vi "updateM300NTCENTwithPeeling.vi"() -> ()   [LabVIEW 2012]
uses:
  <vilib>/addons/database/Connection.llb/DB Tools Open Connec (Path).vi
  <vilib>/addons/database/Connection.llb/Conn Execute.vi
  <vilib>/addons/database/Recordset.llb/Rec Destroy - Connection.vi
  <vilib>/addons/database/Recordset.llb/Rec Fetch Recordset Data (R).vi
  <vilib>/addons/database/_DB Variant To Data/Database Variant To Data.xnode
  <vilib>/addons/database/NI_Database_API.lvlib
panel:
  out "concatenated string":string
  out "error out":errorcluster
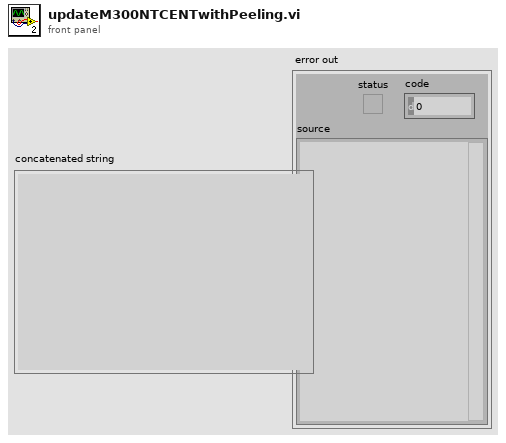
[diagram p1: front panel]
types:
  T1 = typedef "NI_Database_API.lvlib/Conn ObjectReference.ctl" = refnum<k1>
  T2 = typedef "NI_Database_API.lvlib/Rec ObjectReference.ctl" = refnum<k1>
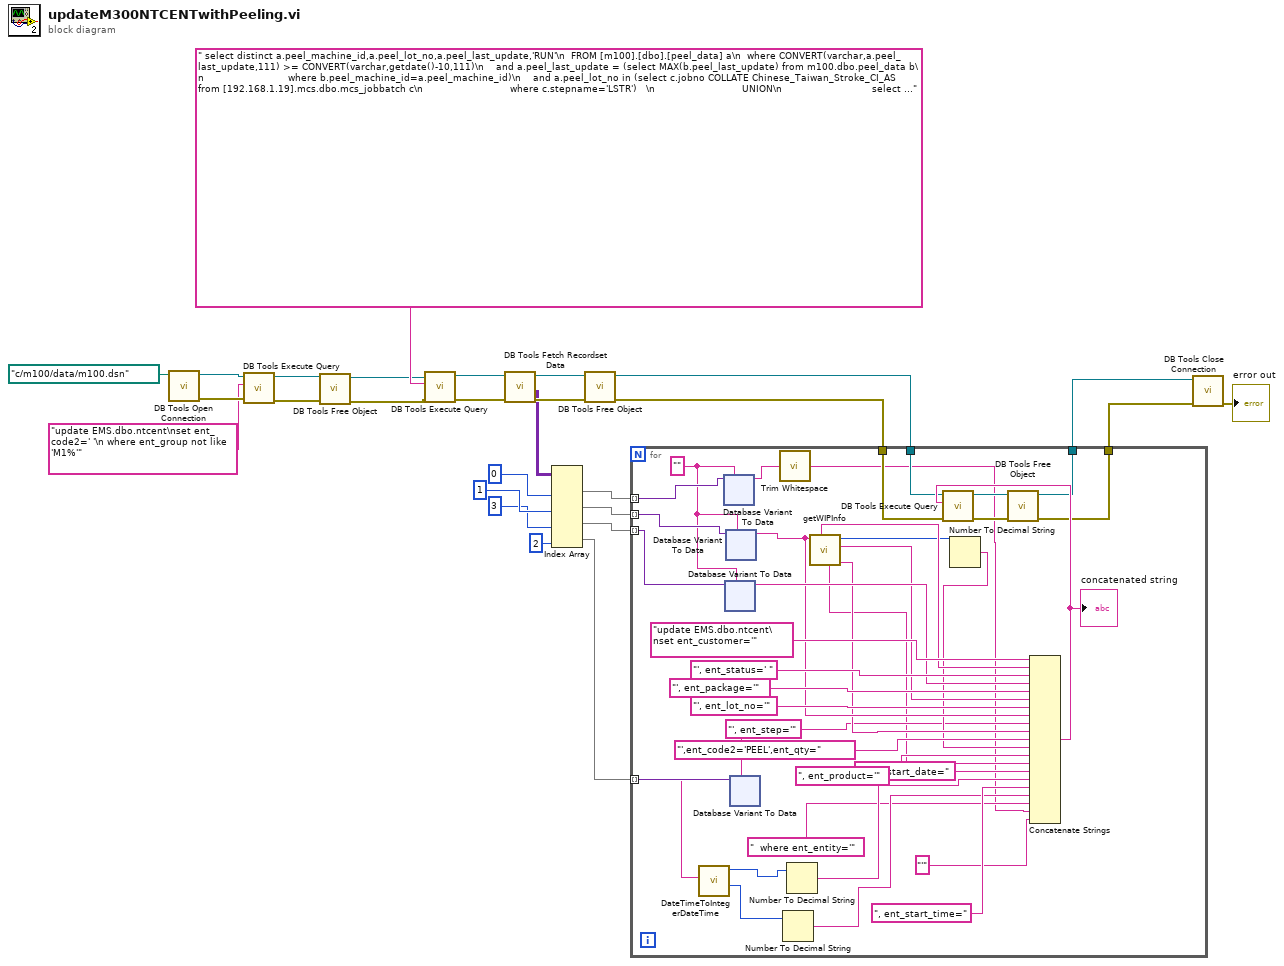
[diagram p0: block diagram]
diagram:
  n1 = call-poly <vilib>:"DB Tools Open Connection.vi"("connection information"=path "c:/m100/data/m100.dsn") -> ("error out"=w4:errorcluster, "connection reference"=w7:T1)  [unwired: 7 in]
  n2 = call-poly <vilib>:"DB Tools Execute Query.vi"("error in (no error)"=w4, "SQL query"="update EMS.dbo.ntcent\nset ent_code2=' '\n where ent_group not like 'M1%'", "connection reference"=w7) -> ("error out"=w3:errorcluster, "recordset reference"=w6:T2)  [unwired: 5 in]
  n3 = call-poly <vilib>:"DB Tools Free Object.vi"("error in (no error)"=w3, "recordset reference"=w6) -> ("error out"=w2:errorcluster, "connection reference"=w5:T1)  [unwired: 8 in]
  n4 = call-poly <vilib>:"DB Tools Execute Query.vi"("error in (no error)"=w2, "SQL query"=" select distinct a.peel_machine_id,a.peel_lot_no,a.peel_last_update,'RUN'\n  FROM [m100].[dbo].[peel_data] a\n  where CONVERT(varchar,a.peel_last_update,111) >= CONVERT(varchar,getdate()-10,111)\n    and a.peel_last_update = (select MAX(b.peel_last_update) from m100.dbo.peel_data b\n                            where b.peel_machine_id=a.peel_machine_id)\n    and a.peel_lot_no in (select c.jobno COLLATE Chinese_Taiwan_Stroke_CI_AS from [192.168.1.19].mcs.dbo.mcs_jobbatch c\n                             where c.stepname='LSTR')   \n                             UNION\n                              select distinct a.peel_machine_id,a.peel_lot_no,a.peel_last_update,'IDLE'\n  FROM [m100].[dbo].[peel_data] a\n  where CONVERT(varchar,a.peel_last_update,111) >= CONVERT(varchar,getdate()-10,111)\n    and a.peel_last_update = (select MAX(b.peel_last_update) from m100.dbo.peel_data b\n                            where b.peel_machine_id=a.peel_machine_id)\n    and a.peel_lot_no NOT in (select c.jobno COLLATE Chinese_Taiwan_Stroke_CI_AS from [192.168.1.19].mcs.dbo.mcs_jobbatch c\n                             where c.stepname='LSTR')  \n  order by a.peel_machine_id", "connection reference"=w5) -> ("error out"=w25:errorcluster, "recordset reference"=w27:T2)  [unwired: 5 in]
  n5 = call-poly <vilib>:"DB Tools Fetch Recordset Data.vi"("error in (no error)"=w25, "recordset reference"=w27) -> ("error out"=w24:errorcluster, "recordset data"=w21:variant[][], "recordset reference out"=w26:T2)  [unwired: 3 in]
  n6 = Index Array(array=w21, index (col) #1=0 ("disabled index (col)"), index (col) #2=1 ("index (col)"), index (col) #3=3 ("index (col)"), index (col) #4=2 ("index (col)")) -> (element #1=w17:variant[], element #2=w16:variant[], element #3=w15:variant[], element #4=w13:variant[])  [unwired: 4 in]
  n7 = call-poly <vilib>:"DB Tools Free Object.vi"("error in (no error)"=w24, "recordset reference"=w26) -> ("error out"=w11:errorcluster, "connection reference"=w12:T1)  [unwired: 8 in]
  n8 = for {
    tunnel: w17 -> [w65] mode=indexing
    tunnel: w16 -> [w64] mode=indexing
    tunnel: w15 -> [w63] mode=indexing
    tunnel: w13 -> [w54] mode=indexing
    tunnel: w12 -> [w52]
    tunnel: w11 -> [w51]
    tunnel: [w48] -> w10
    tunnel: [w47] -> w9
    w40 = "', ent_step='" ("string")
    w62 = ""
    n9 = xnode "Database Variant To Data"("database variant"=w65, "type"=w62) -> ("data"=w46:string)  [unwired: 1 in, 1 out]
    n10 = xnode "Database Variant To Data"("database variant"=w63, "type"=w62) -> ("data"=w58:string)  [unwired: 1 in, 1 out]
    n11 = xnode "Database Variant To Data"("database variant"=w64, "type"=w62) -> ("data"=w45:string)  [unwired: 1 in, 1 out]
    n12 = xnode "Database Variant To Data"("database variant"=w54, "type"=w40) -> ("data"=w37:string)  [unwired: 1 in, 1 out]
    n13 = call "DateTimeToIntegerDateTime.vi"("Datetime string"=w37) -> ("Time"=w35:i32, "Date"=w36:i32)  [unwired: 9 in]
    n14 = call <vilib>:"Trim Whitespace.vi"("string"=w46) -> ("trimmed string"=w29:string)  [unwired: 1 in]
    n15 = Number To Decimal String(number=w35) -> (decimal integer string=w31:string)  [unwired: 1 in]
    n16 = Number To Decimal String(number=w36) -> (decimal integer string=w33:string)  [unwired: 1 in]
    n17 = call "getWIPInfo.vi"("Lotno"=w45) -> ("step"=w44:string, "Package"=w56:string, "data"=w42:i32, "Product"=w38:string, "CustomerID"=w60:string)  [unwired: 4 in, 2 out]
    n18 = Number To Decimal String(number=w42) -> (decimal integer string=w41:string)  [unwired: 1 in]
    n19 = Concatenate Strings("update EMS.dbo.ntcent\nset ent_customer='" ("string"), w60, "', ent_status=' " ("string"), w58, "', ent_package='" ("string"), w56, "', ent_lot_no='" ("string"), w45, w40, w44, "',ent_code2='PEEL',ent_qty=" ("string"), w41, ", ent_product='" ("string"), w38, "',ent_start_date=" ("string"), w33, ", ent_start_time=" ("string"), w31, "  where ent_entity='" ("string"), w29, "'" ("string")) -> (w53:string)
    "concatenated string" <- w53
    n20 = call-poly <vilib>:"DB Tools Execute Query.vi"("error in (no error)"=w51, "SQL query"=w53, "connection reference"=w52) -> ("error out"=w49:errorcluster, "recordset reference"=w50:T2)  [unwired: 5 in]
    n21 = call-poly <vilib>:"DB Tools Free Object.vi"("error in (no error)"=w49, "recordset reference"=w50) -> ("error out"=w47:errorcluster, "connection reference"=w48:T1)  [unwired: 8 in]
  }
  n22 = call <vilib>:"DB Tools Close Connection.vi"("error in (no error)"=w9, "connection reference"=w10) -> ("error out"=→"error out":errorcluster)  [unwired: 5 in]
